vi "Async Main.vi"(8 "error in (no error)":errorcluster, 11 "Variables in":T1={"Process Ref"=refnum, "Comm Ref"=refnum, "Bus Info"={"Name"="", "Overrides?"=FALSE, "XNET Refs"={"Incoming"="", "Outgoing"=""}, "Port Info"={"Port"="", "Baud Rate"=0, "Termination"=0, "CAN I/O Mode"=0, "FD Baud Rate"=0, "Priority"=0, "FD ISO Mode"=0}, "Frames"=variant(cluster{"Convert Session":refnum<k21>, "ID":u32, "Length":i32, "Offset":i32}[] [])}, "Stream Refs"={"Addon"="", "Port"="", "Filter Ref"=refnum, "Default Filter"={"ID Filters"=[], "Direction Filter"=enum."Tx/Rx", "Type Filter"=enum."All"}, "Port Settings"={"Mode"=0, "Baud Rate"=0, "Termination"=0, "FD ISO Mode"=0, "FD Baud Rate"=0}}, "Data Refs"={"Port.Status"=refnum, "Frame.Enable"=refnum, "Frame.Signals"=refnum, "Frame.Overrides"=refnum, "Port.Enable"=refnum}} {"Stream Refs"."Port Settings"."FD ISO Mode" items=["ISO", "Non ISO", "ISO Legacy"]; "Stream Refs"."Port Settings"."Termination" items=["Off", "On"]; "Stream Refs"."Port Settings"."Mode" items=["CAN 2.0", "CAN FD", "CAN FD+BRS"]; "Bus Info"."Port Info"."FD ISO Mode" items=["ISO", "Non ISO", "ISO Legacy"]; "Bus Info"."Port Info"."CAN I/O Mode" items=["CAN 2.0", "CAN FD", "CAN FD+BRS"]; "Bus Info"."Port Info"."Termination" items=["Off", "On"]}) -> (0 "error out":errorcluster, 3 "Variables out":T1={"Process Ref"=refnum, "Comm Ref"=refnum, "Bus Info"={"Name"="", "Overrides?"=FALSE, "XNET Refs"={"Incoming"="", "Outgoing"=""}, "Port Info"={"Port"="", "Baud Rate"=0, "Termination"=0, "CAN I/O Mode"=0, "FD Baud Rate"=0, "Priority"=0, "FD ISO Mode"=0}, "Frames"=variant(cluster{"Convert Session":refnum<k21>, "ID":u32, "Length":i32, "Offset":i32}[] [])}, "Stream Refs"={"Addon"="", "Port"="", "Filter Ref"=refnum, "Default Filter"={"ID Filters"=[], "Direction Filter"=enum."Tx/Rx", "Type Filter"=enum."All"}, "Port Settings"={"Mode"=0, "Baud Rate"=0, "Termination"=0, "FD ISO Mode"=0, "FD Baud Rate"=0}}, "Data Refs"={"Port.Status"=refnum, "Frame.Enable"=refnum, "Frame.Signals"=refnum, "Frame.Overrides"=refnum, "Port.Enable"=refnum}} {"Stream Refs"."Port Settings"."FD ISO Mode" items=["ISO", "Non ISO", "ISO Legacy"]; "Stream Refs"."Port Settings"."Termination" items=["Off", "On"]; "Stream Refs"."Port Settings"."Mode" items=["CAN 2.0", "CAN FD", "CAN FD+BRS"]; "Bus Info"."Port Info"."FD ISO Mode" items=["ISO", "Non ISO", "ISO Legacy"]; "Bus Info"."Port Info"."CAN I/O Mode" items=["CAN 2.0", "CAN FD", "CAN FD+BRS"]; "Bus Info"."Port Info"."Termination" items=["Off", "On"]})   [LabVIEW 2019, in "Ghost Bus Addon Engine.lvlib"]
uses:
  Ghost Bus Addon Engine.lvlib
  Types/RT Frame Settings.ctl
  <vilib>/NI/NIVS Inline Async API/_Data Access Engine/Data Access Engine/Data Access Engine.lvclass
  <vilib>/NI/NIVS Inline Async API/_Data Access Engine/Data Access Engine/Methods/Read.Data.vi
  <vilib>/xnet/xnet.llb/XNET Read (Frame CAN).vi
  <vilib>/xnet/xnet.llb/XNET Convert (Frame CAN to Signal).vi
  <vilib>/xnet/xnet.llb/XNET Convert (Signal to Frame CAN).vi
  <vilib>/xnet/xnet.llb/XNET Write (Frame CAN).vi
  Types/RT XNET Refs.ctl
  Addon Shared/Types/XNET Port Settings.ctl
  Addon Shared/Ghost Bus Addon Shared.lvlib
  Types/RT Bus Settings.ctl
  <vilib>/NI/NI VeriStand Addon Network Comm/Engine/VeriStand Comm.lvclass
  <vilib>/NI/NIVS Inline Async API/_VS Inline Async API/Process/Process.lvclass
  SubModules/CAN-Streaming-Support/Source/Addon/Addon Shared/Types/Type Filter.ctl
  SubModules/CAN-Streaming-Support/Source/Addon/Addon Shared/CAN Stream Support Shared.lvlib
  SubModules/CAN-Streaming-Support/Source/Addon/Addon Shared/Types/Direction Filter.ctl
  SubModules/CAN-Streaming-Support/Source/Addon/Addon Shared/Types/Filter Parameters.ctl
  SubModules/CAN-Streaming-Support/Source/Addon/Addon Engine/Types/Engine Stream Port Settings.ctl
  SubModules/CAN-Streaming-Support/Source/Addon/Addon Engine/CAN Stream Support Engine.lvlib
  SubModules/CAN-Streaming-Support/Source/Addon/Addon Engine/Types/Engine Stream Refs.ctl
  <vilib>/NI/NIVS Inline Async API/_Data Access Engine/Access Type Classes/Read/Read.lvclass
  <vilib>/NI/NIVS Inline Async API/_Data Access Engine/Data Access Engine/Types/Read.DVR.ctl
  <vilib>/NI/NIVS Inline Async API/_Data Access Engine/Access Type Classes/Write/Write.lvclass
  <vilib>/NI/NIVS Inline Async API/_Data Access Engine/Data Access Engine/Types/Write.DVR.ctl
  Types/RT Data Refs.ctl
  Types/RT Async Engine Variables.ctl
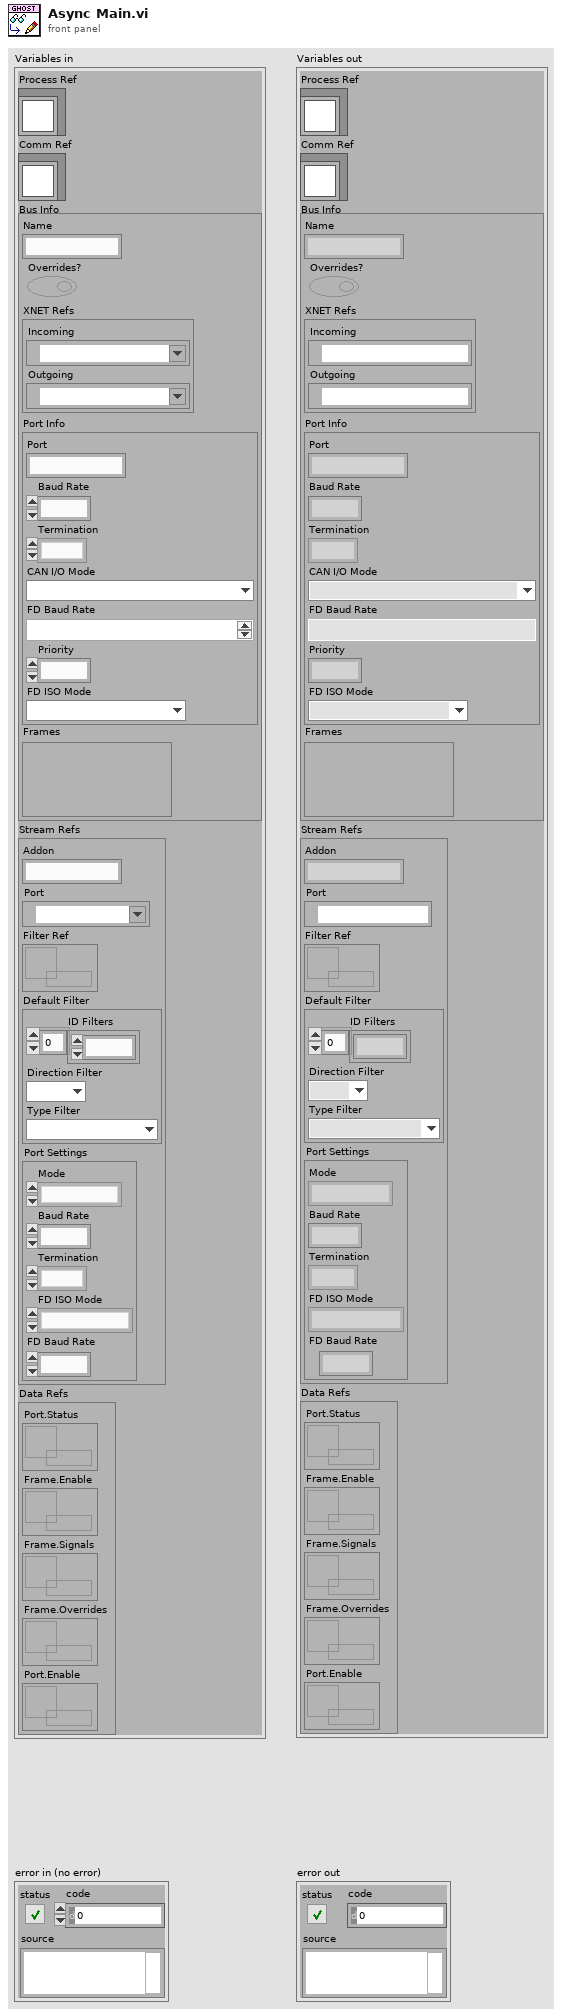
[diagram p1: front panel]
types:
  T1 = typedef "Ghost Bus Addon Engine.lvlib/RT Async Engine Variables.ctl" = cluster{"Process Ref":refnum<class "Process.lvclass">, "Comm Ref":refnum<class "VeriStand Comm.lvclass">, "Bus Info":T2, "Stream Refs":T5, "Data Refs":T10}
  T2 = typedef "RT Bus Settings.ctl" = cluster{"Name":string, "Overrides?":bool, "XNET Refs":T3, "Port Info":T4, "Frames":variant}
  T3 = typedef "Ghost Bus Addon Engine.lvlib/RT XNET Refs.ctl" = cluster{"Incoming":refnum<k21>, "Outgoing":refnum<k21>}
  T4 = typedef "Ghost Bus Addon Shared.lvlib/XNET Port Settings.ctl" = cluster{"Port":string, "Baud Rate":u64, "Termination":u32, "CAN I/O Mode":u32, "FD Baud Rate":u64, "Priority":i32, "FD ISO Mode":u32}
  T5 = typedef "CAN Stream Support Engine.lvlib/Engine Stream Refs.ctl" = cluster{"Addon":string, "Port":refnum<k21>, "Filter Ref":refnum<data-value>, "Default Filter":T6, "Port Settings":T9}
  T6 = typedef "CAN Stream Support Shared.lvlib/Filter Parameters.ctl" = cluster{"ID Filters":u32[], "Direction Filter":T7, "Type Filter":T8}
  T7 = typedef "CAN Stream Support Shared.lvlib/Direction Filter.ctl" = enum16{"Tx/Rx", "Rx", "Tx"}
  T8 = typedef "CAN Stream Support Shared.lvlib/Type Filter.ctl" = enum16{"All", "CAN Data", "CAN Remote", "CAN Bus Error", "CAN 2.0 Data", "CAN FD Data", "CAN FD+BRS Data", "J1939 Data", "Delay", "Log Trigger", "Start Trigger"}
  T9 = typedef "CAN Stream Support Engine.lvlib/Engine Stream Port Settings.ctl" = cluster{"Mode":u32, "Baud Rate":u64, "Termination":u32, "FD ISO Mode":u32, "FD Baud Rate":u64}
  T10 = typedef "Ghost Bus Addon Engine.lvlib/RT Data Refs.ctl" = cluster{"Port.Status":T11, "Frame.Enable":T12, "Frame.Signals":T12, "Frame.Overrides":T12, "Port.Enable":T12}
  T11 = typedef "Data Access Engine.lvlib/Data Access Engine.lvclass/Write.DVR.ctl" = refnum<data-value>
  T12 = typedef "Data Access Engine.lvlib/Data Access Engine.lvclass/Read.DVR.ctl" = refnum<data-value>
  T13 = typedef "Ghost Bus Addon Engine.lvlib/RT Frame Settings.ctl" = cluster{"Convert Session":refnum<k21>, "Length":i32, "Offset":i32, "Enable Offset":i32}
  T14 = typedef "XNET Frame CAN.ctl" = cluster{"timestamp":timestamp, "payload":u8[], "identifier":u32, "type":T15, "extended?":bool, "echo?":bool}
  T15 = typedef "XNET Frame Type CAN.ctl" = u8
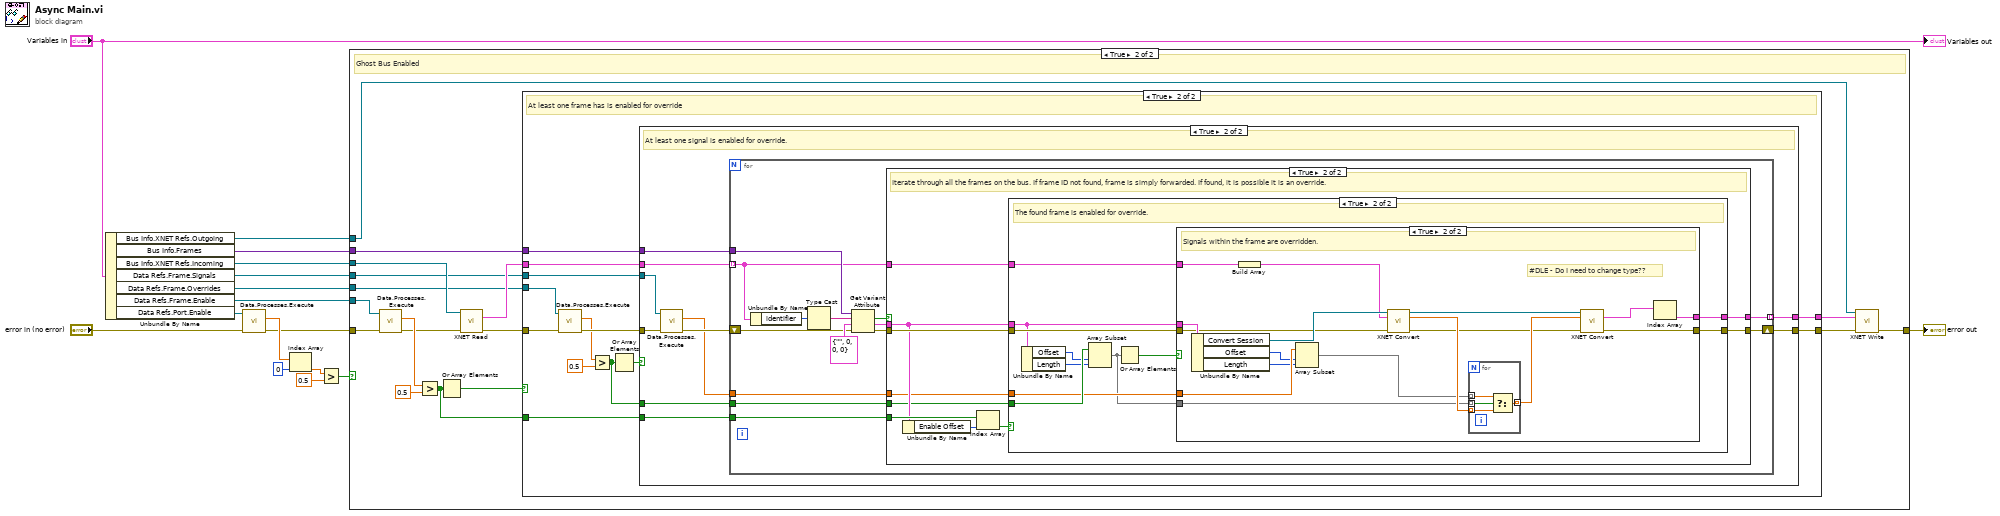
[diagram p0: block diagram]
diagram:
  n1 = Unbundle By Name("Variables in") -> ("Bus Info.XNET Refs.Outgoing"=w3:refnum<k21>, "Bus Info.Frames"=w5:variant, "Bus Info.XNET Refs.Incoming"=w15:refnum<k21>, "Data Refs.Frame.Signals"=w4:T12, "Data Refs.Frame.Overrides"=w6:T12, "Data Refs.Frame.Enable"=w7:T12, "Data Refs.Port.Enable"=w14:T12)
  n2 = call-poly <vilib>:"Data.Processes.Execute.vi"("error in (no error)"="error in (no error)", "Ref"=w14) -> ("error out"=w9:errorcluster, "Values"=w13:dbl[])  [unwired: 7 in, 1 out]
  n3 = Index Array(array=w13, index=0) -> (element=w11:dbl)
  n4 = Greater?(x=w11, y=0.5) -> (0:w8:bool)
  n5 = case shown="True" w8 {
    tunnel: w15 -> [_ w34]
    tunnel: w9 -> [w17 w32]
    tunnel: w7 -> [_ w31]
    tunnel: w3 -> [_ w28]
    tunnel: w6 -> [_ w23]
    tunnel: w5 -> [_ w21]
    tunnel: w4 -> [_ w20]
    tunnel: [w17 w19] -> w1
    frame False {
    }
    frame True {
      # "Ghost Bus Enabled"
      n6 = call-poly <vilib>:"Data.Processes.Execute.vi"("error in (no error)"=w32, "Ref"=w31) -> ("error out"=w22:errorcluster, "Values"=w29:dbl[])  [unwired: 7 in, 1 out]
      n7 = Greater?(x=w29, y=0.5) -> (0:w18:bool[])
      n8 = Or Array Elements(Boolean array=w18) -> (logical OR=w24:bool)
      n9 = call-poly <vilib>:"XNET Read.vi"("session in"=w34, "error in (no error)"=w22) -> ("data"=w33:T14[], "error out"=w27:errorcluster)  [unwired: 10 in, 2 out]
      n10 = case shown="True" w24 {
        tunnel: w33 -> [w35 w49]
        tunnel: w27 -> [w36 w46]
        tunnel: [w36 w43] -> w26
        tunnel: [w35 w42] -> w25
        tunnel: w23 -> [_ w45]
        tunnel: w21 -> [_ w41]
        tunnel: w20 -> [_ w40]
        tunnel: w18 -> [_ w37]
        frame False {
        }
        frame True {
          # "At least one frame has is enabled for override"
          n11 = call-poly <vilib>:"Data.Processes.Execute.vi"("error in (no error)"=w46, "Ref"=w45) -> ("error out"=w47:errorcluster, "Values"=w39:dbl[])  [unwired: 7 in, 1 out]
          n12 = Greater?(x=w39, y=0.5) -> (0:w38:bool[])
          n13 = Or Array Elements(Boolean array=w38) -> (logical OR=w44:bool)
          n14 = case shown="True" w44 {
            tunnel: w49 -> [w50 w61]
            tunnel: w47 -> [w51 w58]
            tunnel: [w51 w59] -> w43
            tunnel: [w50 w53] -> w42
            tunnel: w41 -> [_ w60]
            tunnel: w40 -> [_ w56]
            tunnel: w38 -> [_ w54]
            tunnel: w37 -> [_ w52]
            frame False {
            }
            frame True {
              # "At least one signal is enabled for override."
              n15 = call-poly <vilib>:"Data.Processes.Execute.vi"("error in (no error)"=w58, "Ref"=w56) -> ("error out"=w57:errorcluster, "Values"=w55:dbl[])  [unwired: 7 in, 1 out]
              n16 = for {
                tunnel: w61 -> [w67] mode=indexing
                tunnel: w60 -> [w75]
                shift-right: [w62] -> w59
                shift-left: w57 -> [w71]
                tunnel: w55 -> [w63]
                tunnel: w54 -> [w64]
                tunnel: [w70] -> w53 mode=indexing
                tunnel: w52 -> [w68]
                n17 = Unbundle By Name(w67) -> ("identifier"=w73:u32)
                n18 = Type Cast(x=w73) -> (*(type *) &x=w72:string)  [unwired: 1 in]
                n19 = Get Variant Attribute(Variant=w75, name=w72, default value (empty Variant)=T13 {"Convert Session"="", "Length"=0, "Offset"=0, "Enable Offset"=0} ("cluster"), error in=w71) -> (found=w65:bool, value=w69:T13, error out=w66:errorcluster)  [unwired: 1 out]
                n20 = case shown="True" w65 {
                  tunnel: [w77 w87] -> w70
                  tunnel: w69 -> [_ w81]
                  tunnel: w68 -> [_ w86]
                  tunnel: w67 -> [w77 w83]
                  tunnel: w66 -> [w76 w82]
                  tunnel: w64 -> [_ w80]
                  tunnel: w63 -> [_ w79]
                  tunnel: [w76 w78] -> w62
                  frame False {
                  }
                  frame True {
                    # "Iterate through all the frames on the bus. If frame ID not found, frame is simply forwarded. If found, it is possible it is an override."
                    n21 = Unbundle By Name(w81) -> ("Enable Offset"=w85:i32)
                    n22 = Index Array(array=w86, index=w85) -> (element=w84:bool)
                    n23 = case shown="True" w84 {
                      tunnel: [w89 w100] -> w87
                      tunnel: w83 -> [w89 w95]
                      tunnel: w82 -> [w88 w94]
                      tunnel: w81 -> [_ w92]
                      tunnel: w80 -> [_ w99]
                      tunnel: w79 -> [_ w93]
                      tunnel: [w88 w90] -> w78
                      frame False {
                      }
                      frame True {
                        # "The found frame is enabled for override."
                        n24 = Unbundle By Name(w92) -> ("Offset"=w98:i32, "Length"=w97:i32)
                        n25 = Array Subset(array=w99, index=w98, length=w97) -> (w91:bool[])
                        n26 = Or Array Elements(Boolean array=w91) -> (logical OR=w96:bool)
                        n27 = case shown="True" w96 {
                          tunnel: [w102 w103] -> w100
                          tunnel: w95 -> [w102 w115]
                          tunnel: w94 -> [w101 w113]
                          tunnel: w93 -> [_ w119]
                          tunnel: w92 -> [_ w118]
                          tunnel: w91 -> [_ w109]
                          tunnel: [w101 w104] -> w90
                          frame False {
                          }
                          frame True {
                            # "#DLE - Do I need to change type??"
                            # "Signals within the frame are overridden."
                            n28 = Unbundle By Name(w118) -> ("Convert Session"=w114:refnum<k21>, "Offset"=w117:i32, "Length"=w116:i32)
                            n29 = Build Array(w115) -> (w112:T14[])
                            n30 = Array Subset(array=w119, index=w117, length=w116) -> (w110:dbl[])
                            n31 = call-poly <vilib>:"XNET Convert.vi"("session in"=w114, "frame data"=w112, "error in (no error)"=w113) -> ("session out"=w108:refnum<k21>, "signal data"=w111:dbl[], "error out"=w105:errorcluster)  [unwired: 10 in]
                            n32 = for {
                              tunnel: w111 -> [w121] mode=indexing
                              tunnel: w110 -> [w122] mode=indexing
                              tunnel: w109 -> [w123] mode=indexing
                              tunnel: [w120] -> w107 mode=indexing
                              n33 = Select(t=w122, s=w123, f=w121) -> (s? t:f=w120:dbl)
                            }
                            n34 = call-poly <vilib>:"XNET Convert.vi"("session in"=w108, "signal data"=w107, "error in (no error)"=w105) -> ("frame data"=w106:T14[], "error out"=w104:errorcluster)  [unwired: 9 in, 2 out]
                            n35 = Index Array(array=w106) -> (element=w103:T14)  [unwired: 1 in]
                          }
                        }
                      }
                    }
                  }
                }
              }
            }
          }
        }
      }
      n36 = call-poly <vilib>:"XNET Write.vi"("session in"=w28, "data"=w25, "error in (no error)"=w26) -> ("error out"=w19:errorcluster)  [unwired: 11 in, 1 out]
    }
  }
  "error out" <- w1
  "Variables out" <- "Variables in"
